vi "MouseInput.vi"() -> ()   [LabVIEW 2019]
uses:
  <vilib>/Utility/inputDevices.llb/mouseAcquire.vi
  <vilib>/Utility/inputDevices.llb/closeMouse.vi
panel:
  out "Mouse Position\nCluster":T1={"Horizontal"=280, "Vertical"=230, "Scrolling"=0}
  out "Mouse Button Cluster":cluster{"Left Button":bool, "Right Button":bool}
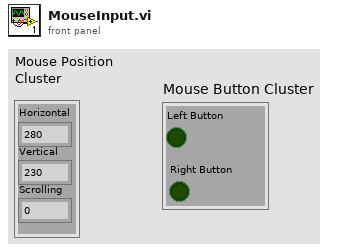
[diagram p1: front panel]
types:
  T1 = cluster{"Horizontal":i32, "Vertical":i32, "Scrolling":i32}
  T2 = cluster{"button 1":bool, "button 2":bool, "button 3":bool, "button 4":bool}
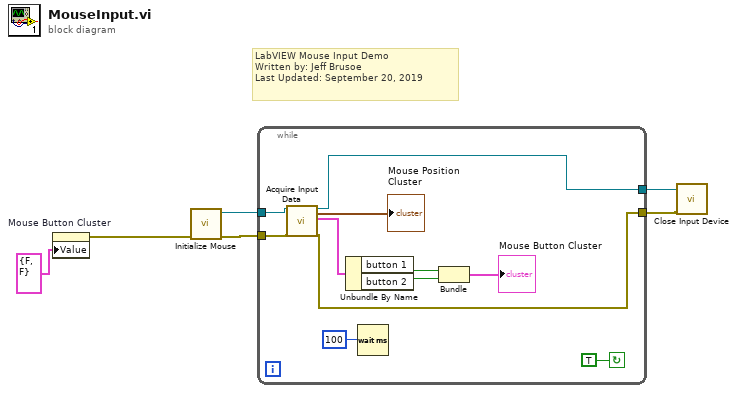
[diagram p0: block diagram]
diagram:
  # "LabVIEW Mouse Input Demo\nWritten by: Jeff Brusoe\nLast Updated: September 20, 2019"
  n1 = property on="Mouse Button Cluster" class="Clust (strict)"("Value"=cluster{bool, bool} {FALSE, FALSE}) -> (error out=w6:errorcluster)  [unwired: 2 in, 1 out]
  n2 = call <vilib>:"Initialize Mouse.vi"("error in (no error)"=w6) -> ("error out"=w3:errorcluster, "device ID"=w4:refnum<k1>)  [unwired: 9 in]
  n3 = while {
    tunnel: w3 -> [w16]
    tunnel: w4 -> [w10]
    tunnel: [w8] -> w2
    tunnel: [w7] -> w1
    stop <- TRUE continue-if-true
    n4 = call-poly <vilib>:"Acquire Input Data.vi"("device ID"=w10, "error in (no error)"=w16) -> ("device ID"=w8:refnum<k1>, "axis info"=→"Mouse Position\nCluster":T1, "button info"=w15:T2, "error out"=w7:errorcluster)  [unwired: 14 in]
    n5 = Unbundle By Name(w15) -> ("button 1"=w14:bool, "button 2"=w13:bool)
    n6 = Wait (ms)(milliseconds to wait=u32 100) -> ()  [unwired: 1 out]
    n7 = Bundle("button 1"=w14, "button 2"=w13) -> (→"Mouse Button Cluster":cluster{"button 1":bool, "button 2":bool})  [unwired: 1 in]
  }
  n8 = call-poly <vilib>:"Close Input Device.vi"("error in (no error)"=w1, "device ID"=w2) -> ()  [unwired: 8 in, 1 out]
